vi "Receive.vi"(11 "jettl Queue Actor in":refnum<class "jettl Queue Actor.lvclass">) -> (3 "jettl Queue Actor out":refnum<class "jettl Queue Actor.lvclass">)   [LabVIEW 2021, in "jettl.lvlib" / "jettl Queue Actor.lvlib" / "jettl Queue Actor.lvclass"]
uses:
  jettl Queue Actor.lvclass
  jettl.lvlib
  Actor/Msg/Msg.lvclass
  State/State/State.lvclass
  C:/git/jettl/src/Actor/Actor/Actor.lvclass
  C:/git/jettl/src/Actor/Msgs/Teardown/Teardown/Teardown.lvclass
  C:/git/jettl/src/Actor/Queue Actor/Queue Actor.lvclass
  C:/git/jettl/src/Actor/Msgs/Create/Create/Create.lvclass
  C:/git/jettl/src/Actor/Msgs/Event Last Ack/Event Last Ack/Event Last Ack.lvclass
  C:/git/jettl/src/Actor/Msgs/Queue Last Ack/Queue Last Ack/Queue Last Ack.lvclass
  C:/git/jettl/src/jettl/jettl Queue Actor/jettl Queue Actor/jettl Queue Actor.lvclass
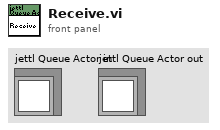
[diagram p1: front panel]
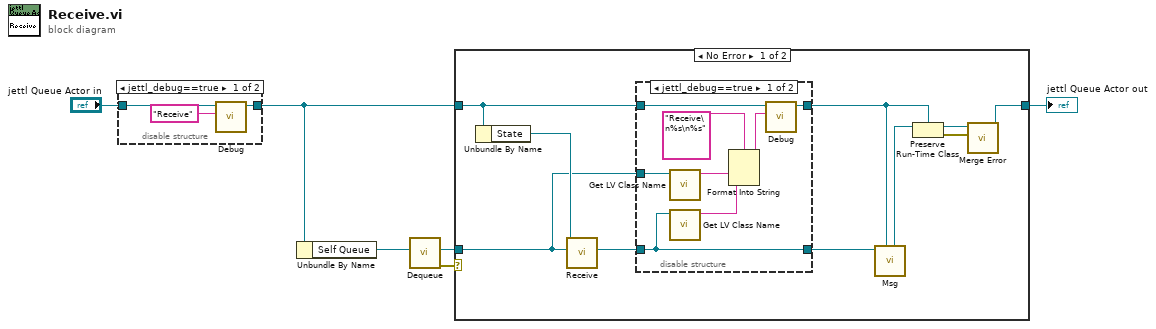
[diagram p0: block diagram]
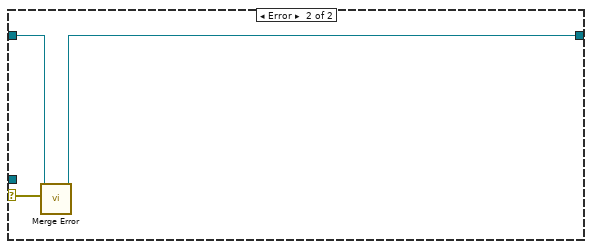
[diagram p4: hidden frame]
diagram:
  n1 = disable-structure shown="jettl_debug==true" {
    disable-tunnel: "jettl Queue Actor in" -> [w9 w10]
    disable-tunnel: [w8 w10] -> w2
    frame condition #0 (active) {
      n2 = call "Debug.vi"("Method"="Receive", "jettl Queue Actor in"=w9) -> ("jettl Queue Actor out"=w8:refnum<class "jettl Queue Actor.lvclass">)  [unwired: 9 in]
    }
    frame condition #1 {
    }
  }
  n3 = Unbundle By Name(w2) -> ("Self Queue"=w6:refnum<data-value>)
  n4 = call "Dequeue.vi"("Queue"=w6) -> ("error out"=w5:errorcluster, "Object"=w4:refnum<class>)  [unwired: 9 in]
  n5 = case shown="No Error" w5 {
    selector: w5 -> [_ w31]
    tunnel: w4 -> [w12 _]
    tunnel: w2 -> [w19 w33]
    tunnel: [w14 w32] -> w1
    frame No Error {
      n6 = Unbundle By Name(w19) -> ("State"=w20:refnum<class "State.lvclass">)
      n7 = call-dynamic "Receive.vi"("Msg in"=w12, "State in"=w20) -> ("Msg out"=w11:refnum<class "Msg.lvclass">)  [unwired: 9 in]
      n8 = disable-structure shown="jettl_debug==true" {
        disable-tunnel: w19 -> [w28 w30]
        disable-tunnel: [w27 w30] -> w16
        disable-tunnel: [w26 w29] -> w17
        disable-tunnel: w11 -> [w26 w29]
        disable-tunnel: w12 -> [w25 _]
        frame condition #0 (active) {
          n9 = call <vilib>:"Get LV Class Name.vi"("object"=w25) -> ("class name"=w24:string)  [unwired: 9 in, 1 out]
          n10 = call <vilib>:"Get LV Class Name.vi"("object"=w26) -> ("class name"=w22:string)  [unwired: 9 in, 1 out]
          n11 = Format Into String(format string="Receive\n%s\n%s" ("Method"), w24, w22) -> (resulting string=w21:string)  [unwired: 2 in, 1 out]
          n12 = call "Debug.vi"("Method"=w21, "jettl Queue Actor in"=w28) -> ("jettl Queue Actor out"=w27:refnum<class "jettl Queue Actor.lvclass">)  [unwired: 9 in]
        }
        frame condition #1 {
        }
      }
      n13 = call-dynamic "Msg.vi"("Actor in"=w16, "Msg in"=w17) -> ("Actor out"=w18:refnum<class "Actor.lvclass">)  [unwired: 9 in]
      n14 = Preserve Run-Time Class(object in=w18, 2:w16) -> (object out=w15:refnum<class "jettl Queue Actor.lvclass">, error out=w13:errorcluster)  [unwired: 1 in]
      n15 = call-dynamic "Merge Error.vi"("Error"=w13, "jettl Queue Actor in"=w15) -> ("jettl Queue Actor out"=w14:refnum<class "jettl Queue Actor.lvclass">)  [unwired: 9 in]
    }
    frame Error {
      n16 = call-dynamic "Merge Error.vi"("Error"=w31, "jettl Queue Actor in"=w33) -> ("jettl Queue Actor out"=w32:refnum<class "jettl Queue Actor.lvclass">)  [unwired: 9 in]
    }
  }
  "jettl Queue Actor out" <- w1
